vi "Controller Drive.vi"   [LabVIEW 2013]
types:
  T1 = typedef "WPI_JoystickButtonState.ctl" = cluster{"Button 1":bool, "Button 2":bool, "Button 3":bool, "Button 4":bool, "Button 5":bool, "Button 6":bool, "Button 7":bool, "Button 8":bool, "Button 9":bool, "Button 10":bool, "Button 11":bool, "Button 12":bool}
  T2 = cluster{"Axes":cluster{"Joystick 1":cluster{"X Axis":dbl, "Y Axis":dbl}, "Triggers":dbl, "Joystick 2":cluster{"X Axis":dbl, "Y Axis":dbl}}, "Buttons":T1}
  T3 = cluster{"Joystick 1":cluster{"X Axis":dbl, "Y Axis":dbl}, "Triggers":dbl, "Joystick 2":cluster{"X Axis":dbl, "Y Axis":dbl}}
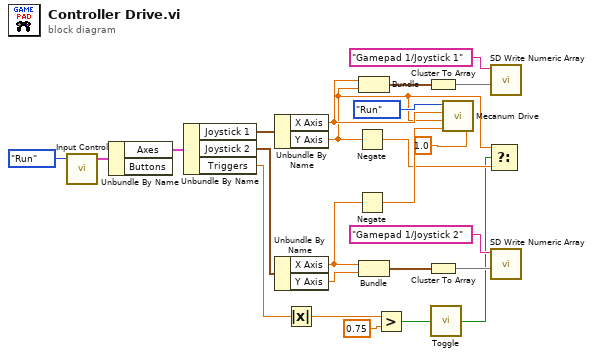
[diagram p0: block diagram]
diagram:
  n1 = call "Input Control.vi"("State"=enum16{"Open", "Run", "End"}."Run") -> ("Gamepad"=w24:T2)  [unwired: 2 in, 2 out]
  n2 = Unbundle By Name(w24) -> ("Axes"=w22:T3)  [unwired: 1 out]
  n3 = Unbundle By Name(w22) -> ("Joystick 1"=w21:cluster{"X Axis":dbl, "Y Axis":dbl}, "Joystick 2"=w11:cluster{"X Axis":dbl, "Y Axis":dbl}, "Triggers"=w5:dbl)
  n4 = Unbundle By Name(w21) -> ("X Axis"=w19:dbl, "Y Axis"=w7:dbl)
  n5 = Unbundle By Name(w11) -> ("X Axis"=w12:dbl, "Y Axis"=w14:dbl)
  n6 = Absolute Value(x=w5) -> (abs(x)=w4:dbl)
  n7 = Negate(x=w7) -> (-x=w6:dbl)
  n8 = Negate(x=w12) -> (-x=w10:dbl)
  n9 = Bundle("X Axis"=w19, "Y Axis"=w7) -> (w8:cluster{"X Axis":dbl, "Y Axis":dbl})  [unwired: 1 in]
  n10 = Bundle("X Axis"=w12, "Y Axis"=w14) -> (w16:cluster{"X Axis":dbl, "Y Axis":dbl})  [unwired: 1 in]
  n11 = Greater?(x=w4, y=0.75) -> (0:w2:bool)
  n12 = Cluster To Array(cluster=w8) -> (array=w18:dbl[])
  n13 = Cluster To Array(cluster=w16) -> (array=w15:dbl[])
  n14 = call "Toggle.vi"("Input"=w2) -> ("Latched"=w1:bool)
  n15 = call "Mecanum Drive.vi"("Division"=1.0, "Turning"=w10, "F/R"=w7, "Strafing"=w19, "State Control"=enum16{"Open", "Run", "End"}."Run") -> ()  [unwired: 3 in]
  n16 = Select(t=w7, s=w1, f=w6) -> ()  [unwired: 1 out]
  n17 = call <vilib>:"SD Write Numeric Array.vi"("Numeric Array"=w18, "Name"="Gamepad 1/Joystick 1") -> ()  [unwired: 8 in, 2 out]
  n18 = call <vilib>:"SD Write Numeric Array.vi"("Numeric Array"=w15, "Name"="Gamepad 1/Joystick 2") -> ()  [unwired: 8 in, 2 out]
